vi "Symphony SetProgPar.vi"(11 "error in":errorcluster) -> (15 "error out":errorcluster)   [LabVIEW 2019]
doc: "Ce Vi enregistre les paramètres des différents axes dans un fichier .ini"
uses:
  <vilib>/Utility/config.llb/Write Key (Boolean).vi
  <vilib>/Utility/config.llb/Write Key (I32).vi
  <vilib>/Utility/config.llb/NI_LVConfig.lvlib
panel:
  in  "X End":i32=1024 min=1 max=1024 step=1
  in  "X Start":i32=1 min=1 max=1024 step=1
  in  "Y Bins":i32=1 min=1 max=256 step=1
  in  "ImageMode":bool
  in  "Launch server":bool=TRUE
  in  "InitOnStart":bool=TRUE
  in  "Shutter Enable":bool=TRUE
  in  "ADC":u16 caption="Device Name"
  in  "Gain":u16=2 caption="Device Name"
  in  "Int_time(ms)":i16=10 caption="Integration time(ms)"
  in  "Accumulations:":u16=1 caption="Accumulations" min=1 step=1
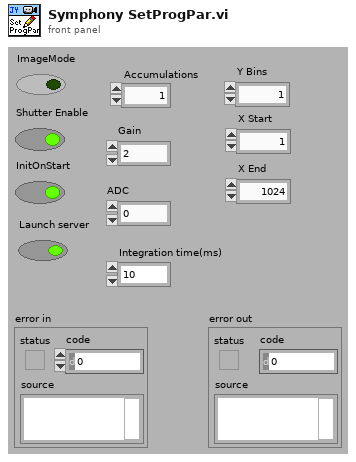
[diagram p1: front panel]
types:
  T1 = typedef "NI_LVConfig.lvlib/Config Data RefNum.ctl" = refnum<k1>
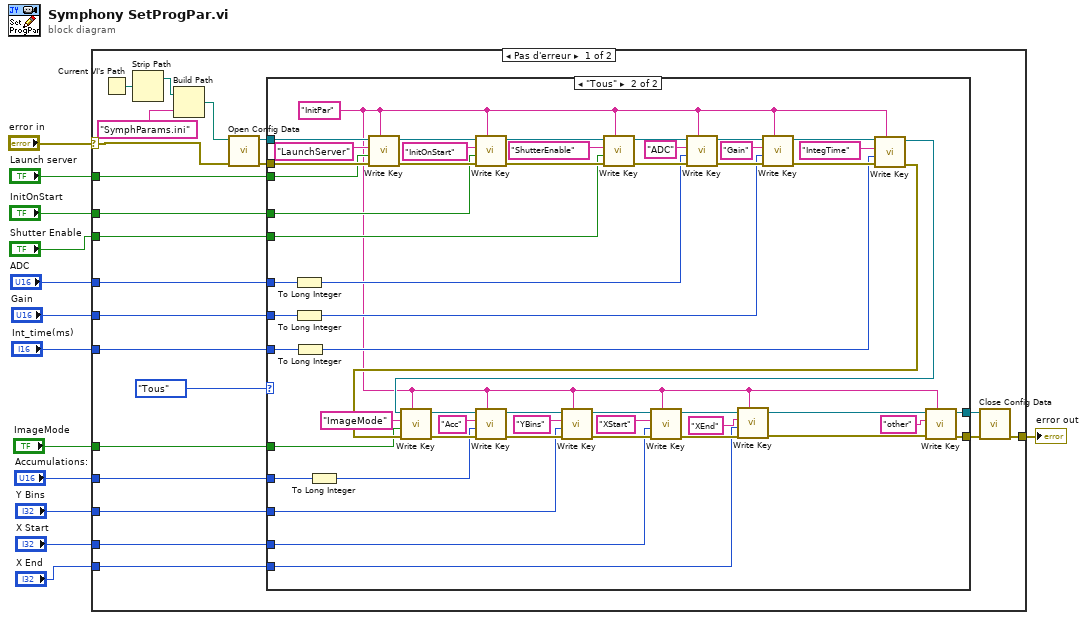
[diagram p0: block diagram]
diagram:
  n1 = case shown="Pas d'erreur" "error in" {
    selector: "error in" -> [w26 w92]
    tunnel: [w30 w92] -> w13
    tunnel: "Launch server" -> [w25 _]
    tunnel: "InitOnStart" -> [w24 _]
    tunnel: "Shutter Enable" -> [w23 _]
    tunnel: "Int_time(ms)" -> [w22 _]
    tunnel: "ADC" -> [w21 _]
    tunnel: "Gain" -> [w20 _]
    tunnel: "ImageMode" -> [w18 _]
    tunnel: "Accumulations:" -> [w17 _]
    tunnel: "Y Bins" -> [w16 _]
    tunnel: "X Start" -> [w15 _]
    tunnel: "X End" -> [w14 _]
    frame No Error {
      n2 = Current VI's Path() -> (path=w35:path)
      n3 = Strip Path(path=w35) -> (stripped path=w27:path)  [unwired: 1 out]
      n4 = Build Path(base path=w27, name or relative path="SymphParams.ini") -> (appended path=w33:path)
      n5 = call <vilib>:"Open Config Data.vi"("error in (no error)"=w26, "configuration file path"=w33) -> ("error out"=w31:errorcluster, "refnum"=w32:T1)  [unwired: 7 in, 1 out]
      n6 = case shown="\"Tous\"" enum16{"One", "Tous"}."Tous" ("Param") {
        tunnel: w32 -> [w37 w83]
        tunnel: w31 -> [w36 w82]
        tunnel: [w36 w55] -> w29
        tunnel: [w37 w54] -> w28
        tunnel: w25 -> [_ w53]
        tunnel: w24 -> [_ w52]
        tunnel: w23 -> [_ w51]
        tunnel: w22 -> [_ w50]
        tunnel: w21 -> [_ w49]
        tunnel: w20 -> [_ w48]
        tunnel: w18 -> [_ w44]
        tunnel: w17 -> [_ w43]
        tunnel: w16 -> [_ w41]
        tunnel: w15 -> [_ w39]
        tunnel: w14 -> [_ w38]
        frame Default {
          # "choix invalide!"
        }
        frame "Tous" {
          w40 = "InitPar" ("section")
          n7 = To Long Integer(number=w49) -> (32bit integer=w47:i32)
          n8 = To Long Integer(number=w48) -> (32bit integer=w46:i32)
          n9 = To Long Integer(number=w50) -> (32bit integer=w45:i32)
          n10 = To Long Integer(number=w43) -> (32bit integer=w42:i32)
          n11 = call-poly <vilib>:"Write Key.vi"("section"=w40, "error in (no error)"=w82, "value"=w53, "key"="LaunchServer", "refnum"=w83) -> ("error out"=w79:errorcluster, "refnum out"=w81:T1)  [unwired: 4 in, 1 out]
          n12 = call-poly <vilib>:"Write Key.vi"("section"=w40, "error in (no error)"=w79, "value"=w52, "key"="InitOnStart", "refnum"=w81) -> ("error out"=w78:errorcluster, "refnum out"=w73:T1)  [unwired: 4 in, 1 out]
          n13 = call-poly <vilib>:"Write Key.vi"("section"=w40, "error in (no error)"=w78, "value"=w51, "key"="ShutterEnable", "refnum"=w73) -> ("error out"=w77:errorcluster, "refnum out"=w74:T1)  [unwired: 4 in, 1 out]
          n14 = call-poly <vilib>:"Write Key.vi"("section"=w40, "error in (no error)"=w77, "value"=w47, "key"="ADC", "refnum"=w74) -> ("error out"=w76:errorcluster, "refnum out"=w75:T1)  [unwired: 4 in, 1 out]
          n15 = call-poly <vilib>:"Write Key.vi"("section"=w40, "error in (no error)"=w76, "value"=w46, "key"="Gain", "refnum"=w75) -> ("error out"=w60:errorcluster, "refnum out"=w59:T1)  [unwired: 4 in, 1 out]
          n16 = call-poly <vilib>:"Write Key.vi"("section"=w40, "error in (no error)"=w60, "value"=w45, "key"="IntegTime", "refnum"=w59) -> ("error out"=w62:errorcluster, "refnum out"=w61:T1)  [unwired: 4 in, 1 out]
          n17 = call-poly <vilib>:"Write Key.vi"("section"=w40, "error in (no error)"=w62, "value"=w44, "key"="ImageMode", "refnum"=w61) -> ("error out"=w71:errorcluster, "refnum out"=w72:T1)  [unwired: 4 in, 1 out]
          n18 = call-poly <vilib>:"Write Key.vi"("section"=w40, "error in (no error)"=w71, "value"=w42, "key"="Acc", "refnum"=w72) -> ("error out"=w69:errorcluster, "refnum out"=w70:T1)  [unwired: 4 in, 1 out]
          n19 = call-poly <vilib>:"Write Key.vi"("section"=w40, "error in (no error)"=w69, "value"=w41, "key"="YBins", "refnum"=w70) -> ("error out"=w67:errorcluster, "refnum out"=w68:T1)  [unwired: 4 in, 1 out]
          n20 = call-poly <vilib>:"Write Key.vi"("section"=w40, "error in (no error)"=w67, "value"=w39, "key"="XStart", "refnum"=w68) -> ("error out"=w66:errorcluster, "refnum out"=w65:T1)  [unwired: 4 in, 1 out]
          n21 = call-poly <vilib>:"Write Key.vi"("section"=w40, "error in (no error)"=w66, "value"=w38, "key"="XEnd", "refnum"=w65) -> ("error out"=w56:errorcluster, "refnum out"=w57:T1)  [unwired: 4 in, 1 out]
          n22 = call-poly <vilib>:"Write Key.vi"("section"=w40, "error in (no error)"=w56, "key"="other", "refnum"=w57) -> ("error out"=w55:errorcluster, "refnum out"=w54:T1)  [unwired: 5 in, 1 out]
        }
      }
      n23 = call <vilib>:"Close Config Data.vi"("error in (no error)"=w29, "refnum"=w28) -> ("error out"=w30:errorcluster)  [unwired: 8 in, 1 out]
    }
    frame Error {
    }
  }
  "error out" <- w13
